vi "GetTotePos.vi"(3 "Bottom Right":cluster{"x":i16, "y":i16}, 4 "Bottom Left":cluster{"x":i16, "y":i16}, 5 "Top Right":cluster{"x":i16, "y":i16}, 6 "Top Left":cluster{"x":i16, "y":i16}) -> (0 "X Offset":dbl=-2.5, 1 "Angle":dbl, 2 "Distance":dbl=15.0)   [LabVIEW 2014]
panel:
  in  "Picking up from side?":bool
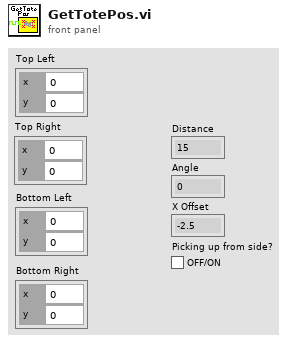
[diagram p1: front panel]
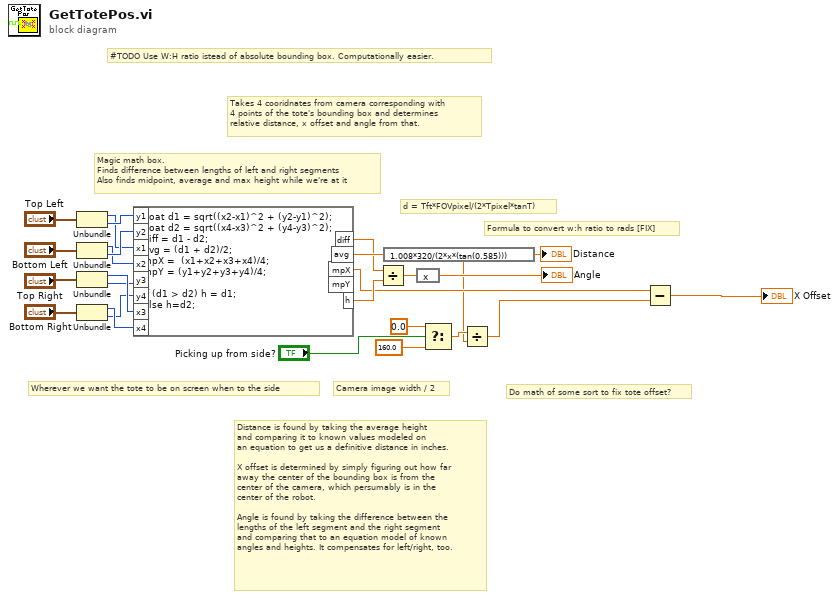
[diagram p0: block diagram]
diagram:
  # "#TODO Use W:H ratio istead of absolute bounding box. Computationally easier."
  # "Do math of some sort to fix tote offset?"
  # "Wherever we want the tote to be on screen when to the side"
  # "Distance is found by taking the average height\nand comparing it to known values modeled on\nan equation to get us a definitive distance in inches.\n\nX offset is determined by simply figuring out how far\naway the center of the bounding box is from the\ncenter of the camera, which persumably is in the\ncenter of the robot.\n\nAngle is found by taking the difference between the\nlengths of the left segment and the right segment\nand comparing that to an equation model of known\nangles and heights. It compensates for left/right, too."
  # "Camera image width / 2"
  # "Formula to convert w:h ratio to rads [FIX]"
  # "d = Tft*FOVpixel/(2*Tpixel*tanT)"
  # "Magic math box.\nFinds difference between lengths of left and right segments\nAlso finds midpoint, average and max height while we're at it"
  # "Takes 4 cooridnates from camera corresponding with\n4 points of the tote's bounding box and determines\nrelative distance, x offset and angle from that."
  n1 = Unbundle("Top Left") -> ("x"=w21:i16, "y"=w23:i16)
  n2 = Unbundle("Bottom Left") -> ("x"=w20:i16, "y"=w22:i16)
  n3 = Unbundle("Top Right") -> ("x"=w17:i16, "y"=w14:i16)
  n4 = Unbundle("Bottom Right") -> ("x"=w16:i16, "y"=w15:i16)
  n5 = formula code="float d1 = sqrt((x2-x1)^2 + (y2-y1)^2);\nfloat d2 = sqrt((x4-x3)^2 + (y4-y3)^2);\ndiff = d1 - d2;\navg = (d1 + d2)/2;\nmpX =  (x1+x2+x3+x4)/4;\nmpY = (y1+y2+y3+y4)/4;\n\nif (d1 > d2) h = d1; \nelse h=d2;"("y1"=w23, "y2"=w22, "x1"=w21, "x2"=w20, "y3"=w14, "y4"=w15, "x3"=w17, "x4"=w16) -> ("diff"=w12:dbl, "mpX"=w8:dbl, "avg"=w13:dbl, "h"=w11:dbl)  [unwired: 1 out]
  n6 = Divide(x=w12, y=w11) -> (x/y=w10:dbl)
  n7 = expression code="1.008*320/(2*x*(tan(0.585)))"(w13) -> (w2:dbl)
  "Distance" <- w2
  n8 = expression code="x"(w10) -> (→"Angle":dbl)
  n9 = Select(t=0.0, s="Picking up from side?", f=160.0 ("y")) -> (s? t:f=w3:dbl)
  n10 = Divide(x=w3, y=w2) -> (x/y=w1:dbl)
  n11 = Subtract(x=w8, y=w1) -> (x-y=→"X Offset":dbl)
